vi "DriveSetSpeedModifer.vi"(11 "SpeedModifer":dbl) -> ()   [LabVIEW 2023]
uses:
  DriveGlobal.vi
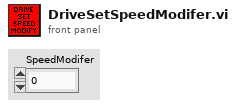
[diagram p1: front panel]
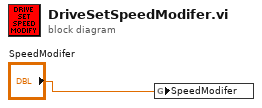
[diagram p0: block diagram]
diagram:
  n1 = global write "DriveGlobal.vi" "SpeedModifer"("SpeedModifer") -> ()
